vi "Parse Record Item by Name.vi"(9 "key":string, 10 "header map in":map{string, i32}(c390), 11 "Record in in":string[](array[string])) -> (0 "found":bool, 1 "Value":string, 2 "header map out":map{string, i32}(c390), 3 "Record out":string[](array[string]))   [LabVIEW 2020, in "Configuration_Helper.lvlib"]
uses:
  Configuration_Helper.lvlib
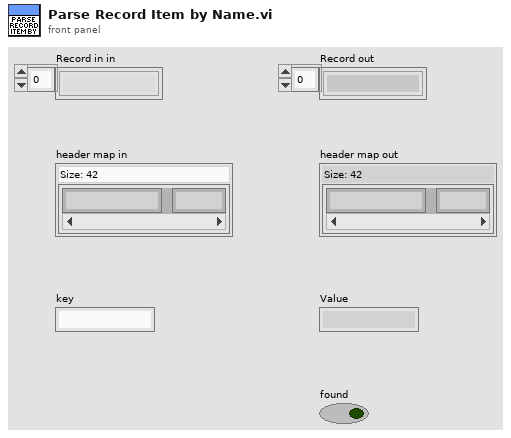
[diagram p1: front panel]
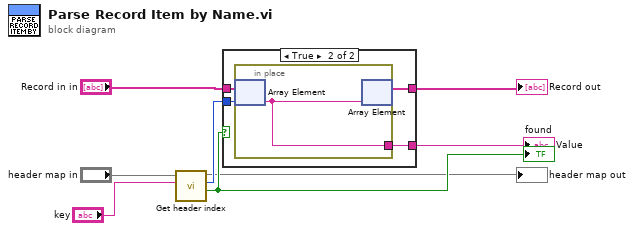
[diagram p0: block diagram]
diagram:
  n1 = call "Get header index.vi"("key"="key", "header map in"="header map in") -> ("found"=w7:bool, "value out"=w5:i32, "header map out"=→"header map out":map{string, i32})  [unwired: 7 in]
  "found" <- w7
  n2 = case shown="True" w7 {
    tunnel: "Record in in" -> [w9 w13]
    tunnel: w5 -> [_ w12]
    tunnel: [_ w11] -> w6
    tunnel: [w9 w10] -> w8
    frame False {
    }
    frame True {
      n3 = in-place {
        in-place-border: [w14] -> w11
        n4 = in-place-array #1(w13, w12) -> (w14:string)
        n5 = in-place-array #1(w14) -> (w10:string[])  [unwired: 1 out]
      }
    }
  }
  "Record out" <- w8
  "Value" <- w6
